vi "PH_Numbers.humanize Value.vi"(2 "Dimension":string, 3 "Round fractional digits (-1)":i16=-1, 4 "Number":dbl) -> (0 "Unit":string, 1 "Value":dbl)   [LabVIEW 2014, in "PH_Common.lvlib"]
doc: "This VI makes a data value readable for human: The ingoing number is set to a digitized value and a Unit with prefix. The VI handels Nummbers between 10^18 ... 10^-15.\n\nExample: \nAn Input of Number: \"0.025\", Dimension: \"Äpfel\" results in\nValue=25, Unit=mÄpfel \n\nRound fractional digits reduces the indicated digits after the comma; -1 does not touch the number while a value starting from 0 reduces it to percent (0), promille (1) and so on."
uses:
  PH_Common.lvlib
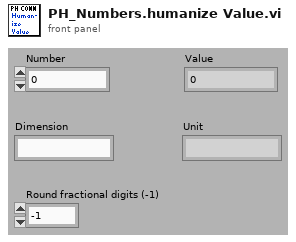
[diagram p1: front panel]
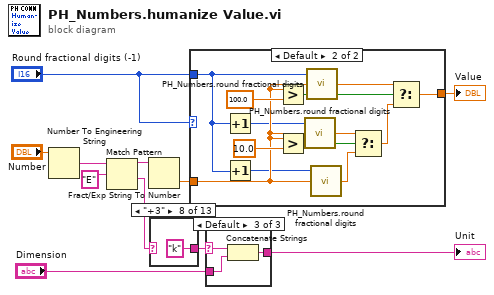
[diagram p0: block diagram]
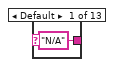
[diagram p5: hidden frame]
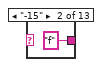
[diagram p6: hidden frame]
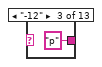
[diagram p7: hidden frame]
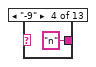
[diagram p8: hidden frame]
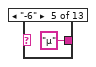
[diagram p9: hidden frame]
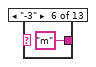
[diagram p10: hidden frame]
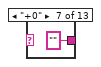
[diagram p11: hidden frame]
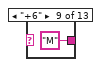
[diagram p12: hidden frame]
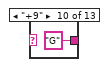
[diagram p13: hidden frame]
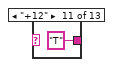
[diagram p14: hidden frame]
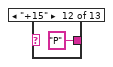
[diagram p15: hidden frame]
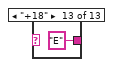
[diagram p16: hidden frame]
diagram:
  n1 = Number To Engineering String(4:"Number") -> (0:w6:string)  [unwired: 3 in]
  n2 = Match Pattern(string=w6, regular expression="E") -> (before substring=w8:string, after substring=w9:string)  [unwired: 1 in, 2 out]
  n3 = Fract/Exp String To Number(string=w8) -> (number=w3:dbl)  [unwired: 3 in, 1 out]
  n4 = case shown="\"+3\"" w9 {
    tunnel: ["N/A" "f" "p" "n" "µ" "m" "" "k" "M" "G" "T" "P" "E"] -> w11
    frame Default {
    }
    frame "-15" {
    }
    frame "-12" {
    }
    frame "-9" {
    }
    frame "-6" {
    }
    frame "-3" {
    }
    frame "+0" {
    }
    frame "+3" {
    }
    frame "+6" {
    }
    frame "+9" {
    }
    frame "+12" {
    }
    frame "+15" {
    }
    frame "+18" {
    }
  }
  n5 = case shown="Default" "Round fractional digits (-1)" {
    tunnel: w3 -> [w25 w30]
    tunnel: [w25 w29] -> w2
    tunnel: "Round fractional digits (-1)" -> [_ w27]
    frame -1 {
    }
    frame Default {
      n6 = Increment(x=w27) -> (x+1=w28:i16)
      n7 = Increment(x=w27) -> (x+1=w26:i16)
      n8 = Greater?(x=w30, y=100.0) -> (0:w37:bool)
      n9 = Greater?(x=w30, y=10.0) -> (0:w34:bool)
      n10 = call "PH_Numbers.round fractional digits.vi"("Input"=w30, "Position (1)"=w28) -> ("round Output"=w33:dbl)
      n11 = call "PH_Numbers.round fractional digits.vi"("Input"=w30, "Position (1)"=w27) -> ("round Output"=w36:dbl)
      n12 = call "PH_Numbers.round fractional digits.vi"("Input"=w30, "Position (1)"=w26) -> ("round Output"=w31:dbl)
      n13 = Select(t=w33, s=w34, f=w31) -> (s? t:f=w32:dbl)
      n14 = Select(t=w36, s=w37, f=w32) -> (s? t:f=w29:dbl)
    }
  }
  "Value" <- w2
  n15 = case shown="Default" w11 {
    selector: w11 -> [w39 _ w42]
    tunnel: [w39 w40 w43] -> w10
    tunnel: "Dimension" -> [_ w40 w41]
    frame "N/A" {
    }
    frame "" {
    }
    frame Default {
      n16 = Concatenate Strings(w42, w41) -> (w43:string)
    }
  }
  "Unit" <- w10
